vi "EXCOM_28.vi"(0 "VISA resource name":refnum<visa-resource-name>, 5 "Error IN":errorcluster) -> (14 "VISA resource name dup":refnum<visa-resource-name>, 15 "NORA":dbl format="%<%H:%M:%S%0u>t", 16 "NODEC":dbl format="%<%H:%M:%S%0u>t", 17 "DEC":dbl format="%.2f", 18 "HA":dbl format="%.2f", 19 "Error OUT":errorcluster)   [LabVIEW 2011]
panel:
  out "RA":dbl format="%<%H:%M:%S%0u>t"
  out "OK Done":bool
  out "Q String":string
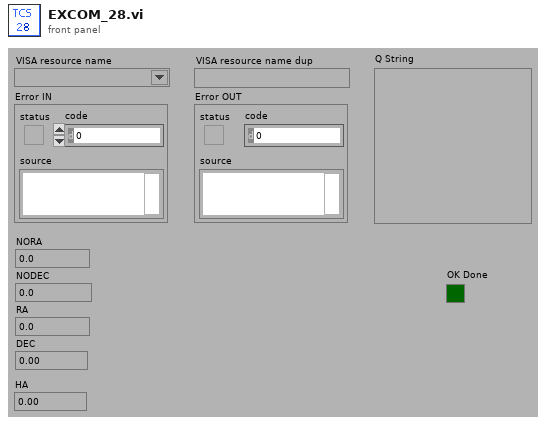
[diagram p1: front panel]
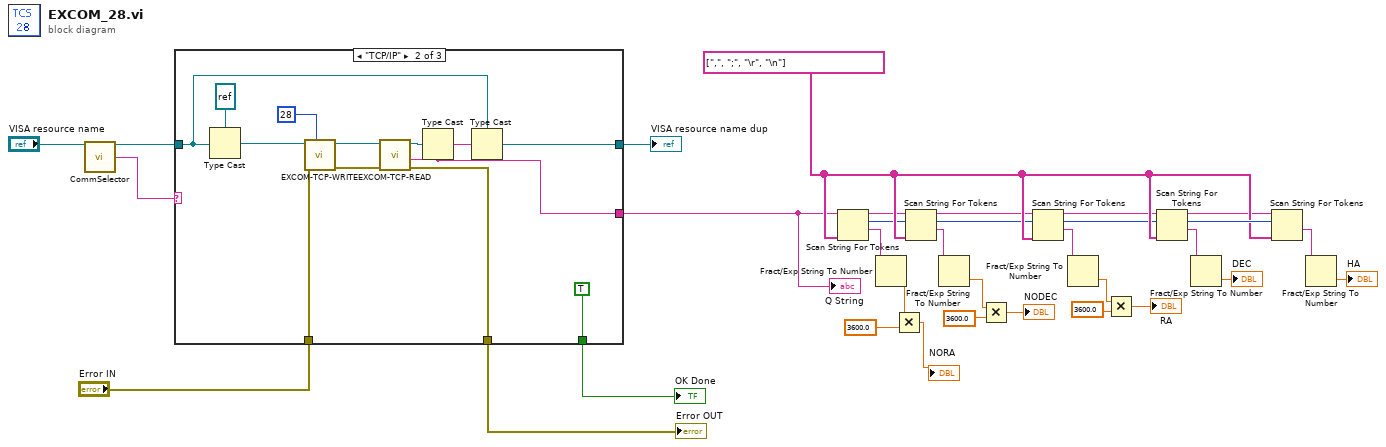
[diagram p0: block diagram]
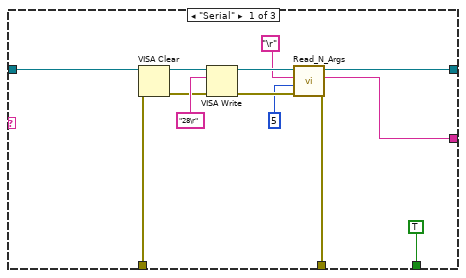
[diagram p2: hidden frame]
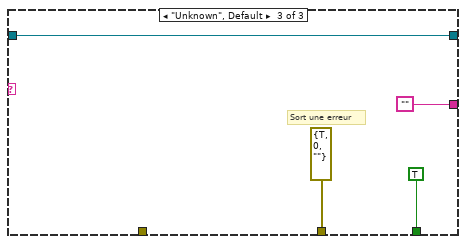
[diagram p3: hidden frame]
diagram:
  w25 = string[] [",", ";", "\r", "\n"] ("delimiters (\\s,\\t,\\r,\\n)")
  n1 = call "CommSelector.vi"("VISA resource name"="VISA resource name") -> ("VISA resource name"=w28:refnum<visa-resource-name>, "CommType"=w27:string)  [unwired: 13 in]
  n2 = case shown="\"TCP/IP\"" w27 {
    tunnel: w28 -> [w38 w49 w61]
    tunnel: [TRUE ("OK Done") TRUE ("OK Done") TRUE ("OK Done")] -> w33
    tunnel: [w45 w53 errorcluster {"status"=TRUE, "code"=0, "source"=""} ("error out")] -> w32
    tunnel: [w39 w48 w61] -> w31
    tunnel: "Error IN" -> [w36 w57 _]
    tunnel: [w34 w51 ""] -> w1
    frame "Serial" {
      n3 = VISA Clear(VISA resource name=w38, error in (no error)=w36) -> (VISA resource name out=w37:refnum<visa-resource-name>, error out=w35:errorcluster)
      n4 = VISA Write(VISA resource name=w37, write buffer="28\r" ("String to Send"), error in (no error)=w35) -> (VISA resource name out=w43:refnum<visa-resource-name>, error out=w44:errorcluster)  [unwired: 1 out]
      n5 = call "Read_N_Args.vi"("Error IN"=w44, "Nb_Args"=5, "Arg_Char"="\r", "VRN IN"=w43) -> ("Error OUT"=w45:errorcluster, "Answer"=w34:string, "VRN OUT"=w39:refnum<visa-resource-name>)  [unwired: 4 in, 1 out]
    }
    frame "TCP/IP" {
      n6 = Type Cast(type=refnum<k5> refnum ("connection ID out"), x=w49) -> (*(type *) &x=w58:refnum<k5>)
      n7 = call "EXCOM-TCP-WRITE.vi"("Commande #"=28, "Error IN"=w57, "connection ID"=w58) -> ("Error OUT"=w54:errorcluster, "connection ID out"=w55:refnum<k5>)  [unwired: 4 in, 2 out]
      n8 = call "EXCOM-TCP-READ.vi"("Error In"=w54, "connection ID"=w55) -> ("Error Out"=w53:errorcluster, "Response"=w51:string, "CID Out"=w52:refnum<k5>)  [unwired: 5 in]
      n9 = Type Cast(type=w51, x=w52) -> (*(type *) &x=w50:string)
      n10 = Type Cast(type=w49, x=w50) -> (*(type *) &x=w48:refnum<visa-resource-name>)
    }
    frame "Unknown", Default {
      # "Sort une erreur"
    }
  }
  "VISA resource name dup" <- w31
  "OK Done" <- w33
  "Error OUT" <- w32
  "Q String" <- w1
  n11 = Scan String For Tokens(6:w25, 9:w1) -> (1:w8:string, 2:w7:i32, 3:w6:string)  [unwired: 4 in, 1 out]
  n12 = Fract/Exp String To Number(string=w8) -> (number=w9:dbl)  [unwired: 3 in, 1 out]
  n13 = Multiply(x=w9, y=3600.0) -> (x*y=→"NORA":dbl)
  n14 = Scan String For Tokens(6:w25, 8:w7, 9:w6) -> (1:w20:string, 2:w4:i32, 3:w5:string)  [unwired: 3 in, 1 out]
  n15 = Fract/Exp String To Number(string=w20) -> (number=w16:dbl)  [unwired: 3 in, 1 out]
  n16 = Multiply(x=w16, y=3600.0) -> (x*y=→"NODEC":dbl)
  n17 = Scan String For Tokens(6:w25, 8:w4, 9:w5) -> (1:w14:string, 2:w2:i32, 3:w3:string)  [unwired: 3 in, 1 out]
  n18 = Fract/Exp String To Number(string=w14) -> (number=w18:dbl)  [unwired: 3 in, 1 out]
  n19 = Multiply(x=w18, y=3600.0) -> (x*y=→"RA":dbl)
  n20 = Scan String For Tokens(6:w25, 8:w2, 9:w3) -> (1:w15:string, 2:w26:i32, 3:w24:string)  [unwired: 3 in, 1 out]
  n21 = Fract/Exp String To Number(string=w15) -> (number=→"DEC":dbl)  [unwired: 3 in, 1 out]
  n22 = Scan String For Tokens(6:w25, 8:w26, 9:w24) -> (1:w23:string)  [unwired: 3 in, 3 out]
  n23 = Fract/Exp String To Number(string=w23) -> (number=→"HA":dbl)  [unwired: 3 in, 1 out]
